vi "Option Parser.vi"(0 "Yokogawa WT1600 in":refnum<class "Yokogawa WT1600.lvclass">, 1 "ID":string, 2 "THD?":bool, 3 "Number of Cards":dbl, 4 "ID cluster.Model":string, 5 "error in (no error)":errorcluster, 7 "Option":string) -> (14 "Yokogawa WT1600 out":refnum<class "Yokogawa WT1600.lvclass">, 19 "error out":errorcluster)   [LabVIEW 2014, in "Generic Power Analyzer.lvlib" / "Yokogawa WT1600.lvlib" / "Yokogawa WT1600.lvclass"]
uses:
  Yokogawa WT1600.lvclass
  <vilib>/regexp/Match Regular Expression.xnode
panel:
  out "Array":string[](array[string])
  out "All cards config":string
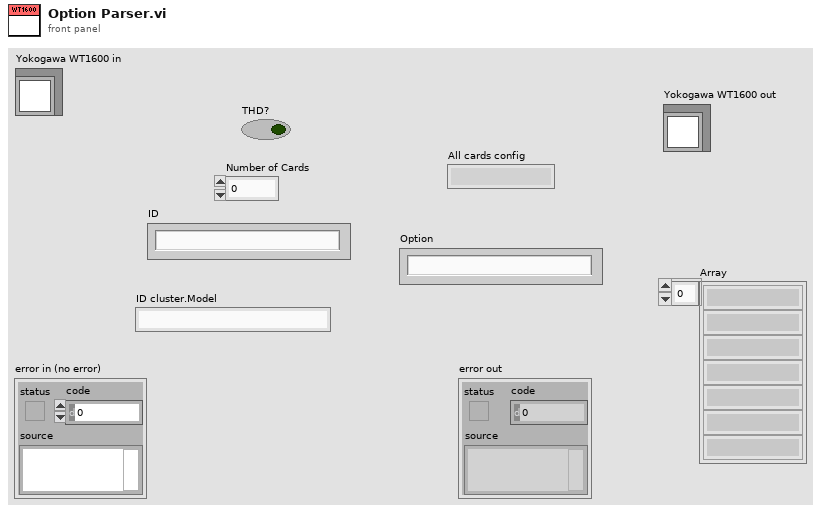
[diagram p1: front panel]
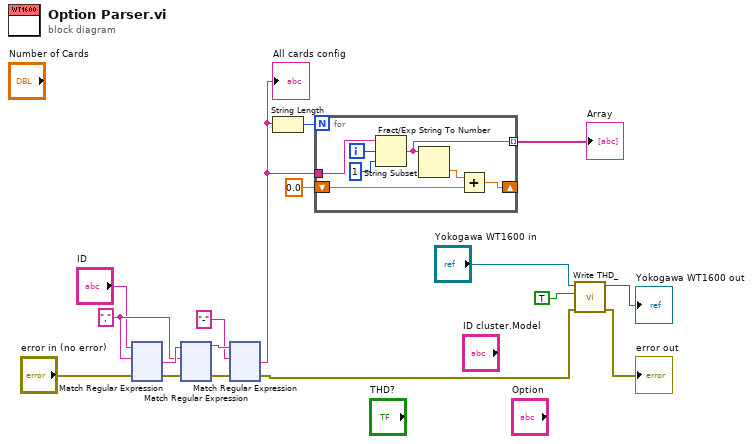
[diagram p0: block diagram]
diagram:
  w16 = "," ("regular expression")
  n1 = xnode "Match Regular Expression"("input string"="ID", "regular expression"=w16, "error in"="error in (no error)") -> ("after match"=w17:string, "error out"=w15:errorcluster)  [unwired: 3 in, 3 out]
  n2 = xnode "Match Regular Expression"("input string"=w17, "regular expression"=w16, "error in"=w15) -> ("before match"=w14:string, "error out"=w12:errorcluster)  [unwired: 3 in, 3 out]
  n3 = xnode "Match Regular Expression"("input string"=w14, "regular expression"="-", "error in"=w12) -> ("after match"=w10:string, "error out"=w2:errorcluster)  [unwired: 3 in, 3 out]
  "All cards config" <- w10
  n4 = String Length(string=w10) -> (length=w11:i32)
  n5 = for {
    N: w11 -> [_]
    tunnel: w10 -> [w24]
    tunnel: [w21] -> w9 mode=indexing
    shift-right: [w18] -> _
    shift-left: 0.0 -> [w19]
    i -> [w23]
    n6 = String Subset(string=w24, offset (0)=w23, length (rest)=1 ("length (rest)")) -> (substring=w21:string)
    n7 = Fract/Exp String To Number(string=w21) -> (number=w20:dbl)  [unwired: 3 in, 1 out]
    n8 = Add(x=w20, y=w19) -> (x+y=w18:dbl)
  }
  "Array" <- w9
  n9 = call-dynamic "Write THD_.vi"("error in (no error)"=w2, "THD?"=TRUE, "Generic Power Analyzer in"="Yokogawa WT1600 in") -> ("error out"=→"error out":errorcluster, "Generic Power Analyzer out"=→"Yokogawa WT1600 out":refnum<class "Yokogawa WT1600.lvclass">)  [unwired: 7 in]
